vi "wave-teste.vi"() -> ()   [LabVIEW 2014]
panel:
  out "mean tf/ti":dbl=0.08694050262673492 format="%0.2f"
  out "number of samples":i32=10
  out "Waveform Graph":dbl[][](graph)
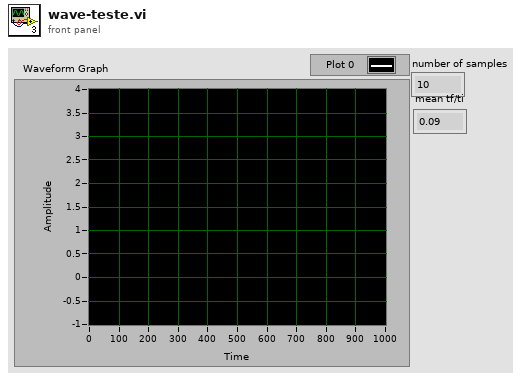
[diagram p1: front panel]
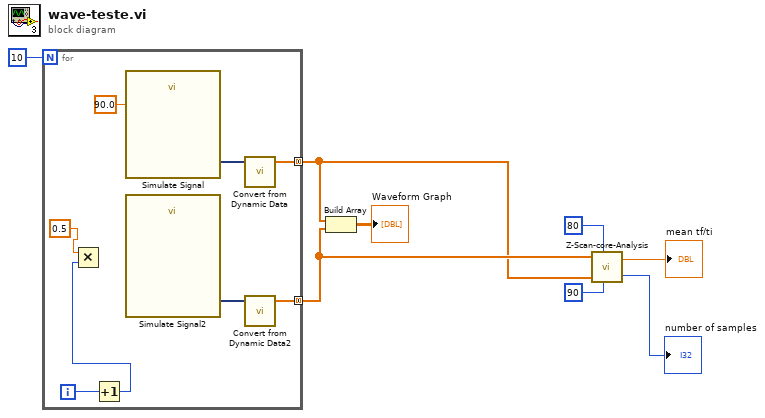
[diagram p0: block diagram]
diagram:
  n1 = for {
    N: 10 -> [_]
    tunnel: [w14] -> w5 mode=concatenating
    tunnel: [w13] -> w6 mode=concatenating
    i -> [w12]
    n2 = Increment(x=w12) -> (x+1=w11:i32)
    n3 = Multiply(x=0.5, y=w11) -> ()  [unwired: 1 out]
    n4 = call "Simulate Signal"("Phase"=90.0) -> ("Square"=w15:dynamicdata)  [unwired: 13 in, 1 out]
    n5 = call "Simulate Signal2"() -> ("Square"=w16:dynamicdata)  [unwired: 14 in, 1 out]
    n6 = call "Convert from Dynamic Data"("Dynamic Data Type"=w15) -> ("Array"=w14:dbl[])  [unwired: 3 in]
    n7 = call "Convert from Dynamic Data2"("Dynamic Data Type"=w16) -> ("Array"=w13:dbl[])  [unwired: 3 in]
  }
  n8 = Build Array(w5, w6) -> (→"Waveform Graph":dbl[][])
  n9 = call "Z-Scan-core-Analysis.vi"("trigger in"=w6, "ti"=80, "signal in"=w5, "tf"=90) -> ("mean tf/ti"=→"mean tf/ti":dbl, "number of samples"=→"number of samples":i32)  [unwired: 1 in]
